vi "Fetch Multi Eval Meas List Segment SEM Results.vi"(7 "Segment (1)":T2=1, 8 "error in (no error)":errorcluster, 9 "Result Type (Current)":i32(ring) items=["Current", "Average", "Extreme", "Standard Deviation"], 10 "Instance (1)":T3=1, 11 "VISA resource name":refnum<visa-resource-name>) -> (0 "error out":errorcluster, 1 "SEM Results":cluster{"OBW":dbl, "TX Power":dbl} {"TX Power" format="%^.3e"; "OBW" format="%^.3e"}, 2 "Reliability Results":T1, 3 "VISA resource name out":refnum<visa-resource-name>, 4 "Statistic Expired":i32, 5 "Out Of Tolerance":dbl format="%^.3e")   [LabVIEW 2020, in "Rohde&Schwarz CMXP NR FR2 Measurement.lvlib"]
doc: "Returns spectrum emission single value results for segment <no> in list mode.\n\nAttributes:\nRSCMXPNRFR2M_ATTR_FETCH_MULTI_EVAL_MEASUREMENT_LIST_SEGMENT_SEM_CURRENT_RESULTS\nRSCMXPNRFR2M_ATTR_FETCH_MULTI_EVAL_MEASUREMENT_LIST_SEGMENT_SEM_AVERAGE_RESULTS\nRSCMXPNRFR2M_ATTR_FETCH_MULTI_EVAL_MEASUREMENT_LIST_SEGMENT_SEM_EXTREME_RESULTS\nRSCMXPNRFR2M_ATTR_FETCH_MULTI_EVAL_MEASUREMENT_LIST_SEGMENT_SEM_STANDARD_DEVIATION_RESULTS\n\nRemote-control commands:\nFETCh:NRMMw:MEAS<i>:MEValuation:LIST:SEGMent<no>:SEMask:CURRent?\nFETCh:NRMMw:MEAS<i>:MEValuation:LIST:SEGMent<no>:SEMask:AVERage?\nFETCh:NRMMw:MEAS<i>:MEValuation:LIST:SEGMent<no>:SEMask:EXTReme?\nFETCh:NRMMw:MEAS<i>:MEValuation:LIST:SEGMent<no>:SEMask:SDEViation?"
uses:
  <instrlib>/Rohde&Schwarz CMXP NR FR2 Measurement/Rohde&Schwarz CMXP NR FR2 Measurement.lvlib
  <instrlib>/Rohde&Schwarz CMXP NR FR2 Measurement/Private/_Instance.ctl
  <instrlib>/Rohde&Schwarz CMXP NR FR2 Measurement/Private/_Segment.ctl
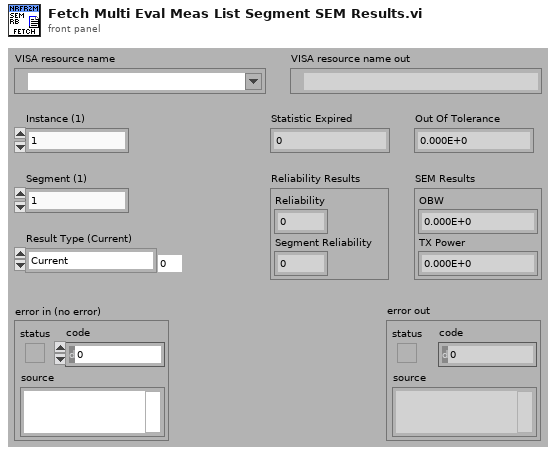
[diagram p1: front panel]
types:
  T1 = cluster{"Reliability":i32, "Segment Reliability":i32}
  T2 = typedef "Rohde&Schwarz CMXP NR FR2 Measurement.lvlib/_Segment.ctl" = i32
  T3 = typedef "Rohde&Schwarz CMXP NR FR2 Measurement.lvlib/_Instance.ctl" = i32
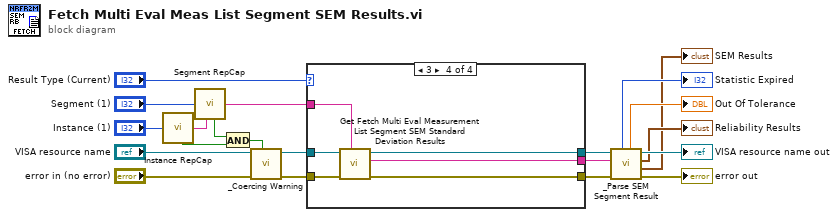
[diagram p0: block diagram]
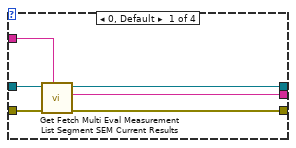
[diagram p2: hidden frame]
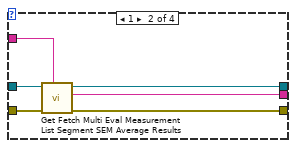
[diagram p3: hidden frame]
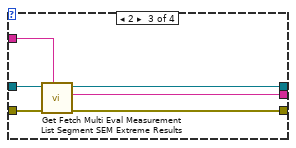
[diagram p4: hidden frame]
diagram:
  n1 = call <instrlib>:"Instance RepCap.vi"("Instance In"="Instance (1)") -> ("In Range?"=w19:bool, "RepCap Identifier Out"=w1:string)  [unwired: 1 in]
  n2 = call <instrlib>:"Segment RepCap.vi"("Segment In"="Segment (1)", "RepCap String In (\"\")"=w1) -> ("In Range?"=w20:bool, "RepCap Identifier Out"=w13:string)
  n3 = And(x=w20, y=w19) -> (x .and. y?=w21:bool)
  n4 = call <instrlib>:"_Coercing Warning.vi"("In Range?"=w21, "error in (no error)"="error in (no error)", "VISA resource name"="VISA resource name") -> ("error out"=w15:errorcluster, "VISA resource name out"=w14:refnum<visa-resource-name>)  [unwired: 7 in]
  n5 = case shown="3" "Result Type (Current)" {
    tunnel: w15 -> [w27 w33 w39 w45]
    tunnel: w14 -> [w26 w32 w38 w44]
    tunnel: w13 -> [w25 w31 w37 w43]
    tunnel: [w24 w30 w36 w42] -> w11
    tunnel: [w23 w29 w35 w41] -> w10
    tunnel: [w22 w28 w34 w40] -> w9
    frame 0, Default {
      n6 = call "Get Fetch Multi Eval Measurement List Segment SEM Current Results"("Repeated Capabilities"=w25, "error in (no error)"=w27, "instrument handle"=w26) -> ("error out"=w24:errorcluster, "Fetch Multi Eval Measurement List Segment SEM Current Results"=w23:string, "instrument handle out"=w22:refnum<visa-resource-name>)  [unwired: 6 in]
    }
    frame 1 {
      n7 = call "Get Fetch Multi Eval Measurement List Segment SEM Average Results"("Repeated Capabilities"=w31, "error in (no error)"=w33, "instrument handle"=w32) -> ("error out"=w30:errorcluster, "Fetch Multi Eval Measurement List Segment SEM Average Results"=w29:string, "instrument handle out"=w28:refnum<visa-resource-name>)  [unwired: 6 in]
    }
    frame 2 {
      n8 = call "Get Fetch Multi Eval Measurement List Segment SEM Extreme Results"("Repeated Capabilities"=w37, "error in (no error)"=w39, "instrument handle"=w38) -> ("error out"=w36:errorcluster, "Fetch Multi Eval Measurement List Segment SEM Extreme Results"=w35:string, "instrument handle out"=w34:refnum<visa-resource-name>)  [unwired: 6 in]
    }
    frame 3 {
      n9 = call "Get Fetch Multi Eval Measurement List Segment SEM Standard Deviation Results"("Repeated Capabilities"=w43, "error in (no error)"=w45, "instrument handle"=w44) -> ("error out"=w42:errorcluster, "Fetch Multi Eval Measurement List Segment SEM Standard Deviation Results"=w41:string, "instrument handle out"=w40:refnum<visa-resource-name>)  [unwired: 6 in]
    }
  }
  n10 = call <instrlib>:"_Parse SEM Segment Result.vi"("error in (no error)"=w11, "Input String"=w10, "VISA resource name"=w9) -> ("error out"=→"error out":errorcluster, "SEM Results"=→"SEM Results":cluster{"OBW":dbl, "TX Power":dbl}, "Reliability Results"=→"Reliability Results":T1, "VISA resource name out"=→"VISA resource name out":refnum<visa-resource-name>, "Out Of Tolerance"=→"Out Of Tolerance":dbl, "Statistic Expired"=→"Statistic Expired":i32)  [unwired: 3 in]
